vi "reverse calibrate.vi"(8 "error in":errorcluster, 10 "Energy Max":dbl, 11 "Energy Min":dbl) -> (0 "error out":errorcluster, 2 "Channel Max":dbl, 3 "Channel Min":dbl)   [LabVIEW 2023]
uses:
  control/param_calibrazione.ctl
panel:
  in  "Calibration":T1
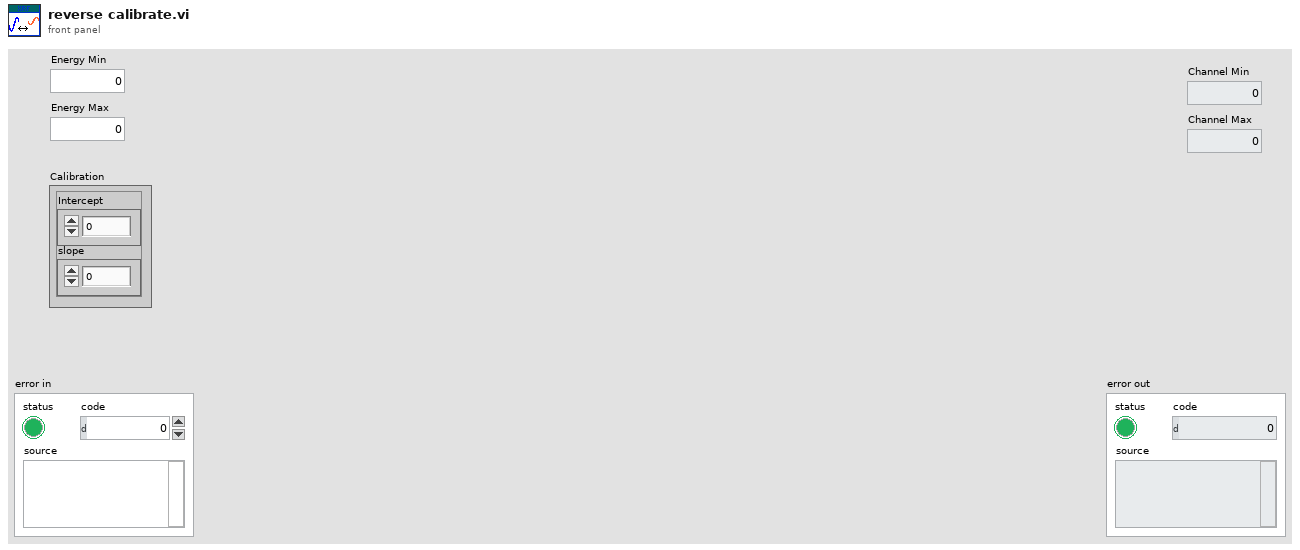
[diagram p1: front panel]
types:
  T1 = typedef "param_calibrazione.ctl" = cluster{"Intercept":dbl, "slope":dbl}
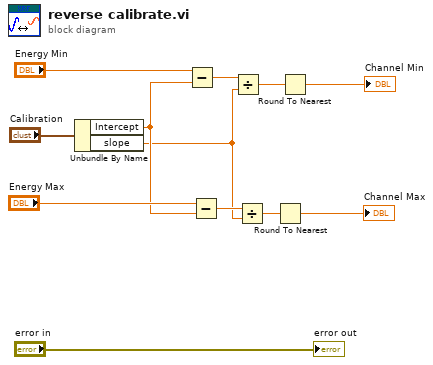
[diagram p0: block diagram]
diagram:
  n1 = Unbundle By Name("Calibration") -> ("Intercept"=w8:dbl, "slope"=w5:dbl)
  n2 = Subtract(x="Energy Min", y=w8) -> (x-y=w7:dbl)
  n3 = Subtract(x="Energy Max", y=w8) -> (x-y=w6:dbl)
  n4 = Divide(x=w7, y=w5) -> (x/y=w3:dbl)
  n5 = Divide(x=w6, y=w5) -> (x/y=w4:dbl)
  n6 = Round To Nearest(number=w4) -> (nearest integer value=→"Channel Max":dbl)
  n7 = Round To Nearest(number=w3) -> (nearest integer value=→"Channel Min":dbl)
  "error out" <- "error in"
